vi "Part B.vi"() -> ()   [LabVIEW 2020]
uses:
  <vilib>/MakerHub/LINX/Public/Peripherals/Analog/Analog Read 1 Chan.vi
  <vilib>/MakerHub/LINX/Public/Peripherals/Digital/Digital Write N Chans.vi
  <vilib>/MakerHub/LINX/Public/Peripherals/Analog/Analog Read N Chans.vi
  <vilib>/MakerHub/LINX/Private/Local IO/LinxDigitalWrite.vi
  <vilib>/MakerHub/LINX/Public/Utilities/Check Channel.vi
  <vilib>/MakerHub/LINX/Private/Local IO/LinxAnalogRead.vi
  <vilib>/MakerHub/LINX/Public/Utilities/Open Serial.vi
  <vilib>/MakerHub/LINX/Private/Utilties/Generate Error.vi
  <vilib>/MakerHub/LINX/LMH-LINX.lvlib
panel:
  in  "?":bool
  out "Temp (C)":dbl(slide) scale=13.0..39.0
  out "Resistance of\nThermistor":dbl
  out "Voltage":dbl
  in  "Analog Channel":u8
  in  "Serial Port":refnum<visa-resource-name>="N/A"
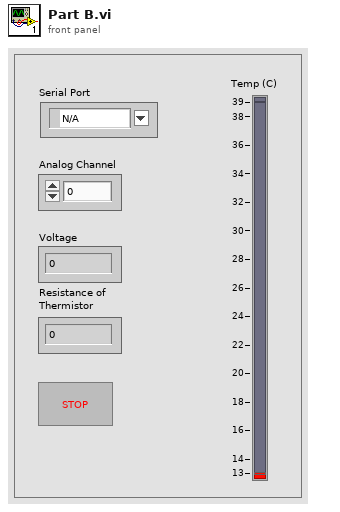
[diagram p1: front panel]
types:
  T1 = typedef "LMH-LINX.lvlib/LINX Ref.ctl" = cluster{"IO":T2, "Interface":T3, "LINX Device Config":T4}
  T2 = typedef "LMH-LINX.lvlib/Platform.ctl" = enum16{"Remote", "Local"}
  T3 = typedef "LMH-LINX.lvlib/Interface.ctl" = enum16{"Serial", "TCP"}
  T4 = typedef "LMH-LINX.lvlib/Device.lvlib/LINX Device Config.ctl" = cluster{"Interface":T3, "COM Port":refnum<visa-resource-name>, "TCP Configuration":T5, "Device Family":u8, "Device ID":u8, "Device Name":string, "TCP Ref":refnum<k5>, "Channels":T6}
  T5 = typedef "LMH-LINX.lvlib/Device.lvlib/TCP Config.ctl" = cluster{"IP Address":string, "Port":u16}
  T6 = typedef "LMH-LINX.lvlib/Channels.ctl" = cluster{"DI":u8[], "DO":u8[], "AI":u8[], "AO":u8[], "PWM":u8[], "QE":u8[], "UART":u8[], "I2C 2":u8[], "SPI":u8[], "CAN":u8[], "Servo":u8[], "AI Ref (V)":dbl, "AI Resolution (Bits)":u8, "AO Ref (V)":dbl, "AO Resolution (Bits)":u8}
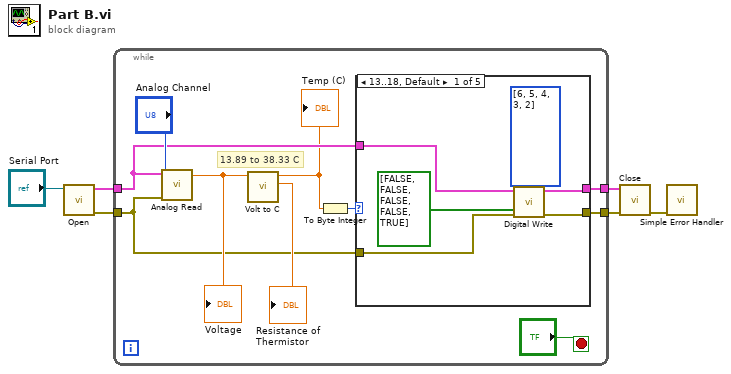
[diagram p0: block diagram]
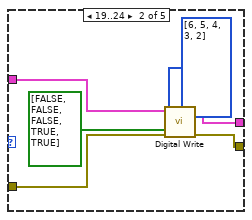
[diagram p2: hidden frame]
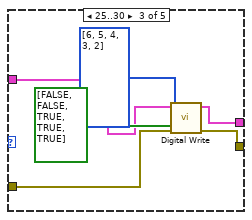
[diagram p3: hidden frame]
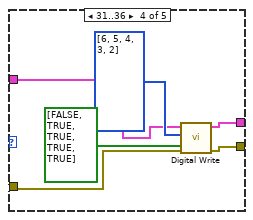
[diagram p4: hidden frame]
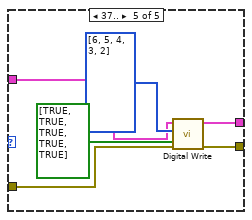
[diagram p5: hidden frame]
diagram:
  n1 = call-poly <vilib>:"Open.vi"("Serial Port"="Serial Port") -> ("Error Out"=w4:errorcluster, "LINX Resource"=w5:T1)  [unwired: 8 in, 1 out]
  n2 = while {
    tunnel: w5 -> [w12]
    tunnel: [w9] -> w2
    tunnel: w4 -> [w11]
    tunnel: [w8] -> w1
    stop <- "?" stop-if-true
    # "13.89 to 38.33 C"
    n3 = call-poly <vilib>:"Analog Read.vi"("Error In"=w11, "Analog Channel"="Analog Channel", "LINX Resource"=w12) -> ("Voltage"=w15:dbl)  [unwired: 5 in, 3 out]
    "Voltage" <- w15
    n4 = call "Volt to C.vi"("Voltage"=w15) -> ("R (ohm)"=→"Resistance of\nThermistor":dbl, "interpolation value"=w10:dbl)  [unwired: 9 in]
    "Temp (C)" <- w10
    n5 = To Byte Integer(number=w10) -> (8bit integer=w13:i8)
    n6 = case shown="13..18, Default" w13 {
      tunnel: [w21 w28 w33 w39 w45] -> w9
      tunnel: [w20 w27 w32 w38 w44] -> w8
      tunnel: w12 -> [w18 w24 w30 w36 w42]
      tunnel: w11 -> [w17 w23 w29 w35 w41]
      frame 13..18, Default {
        n7 = call-poly <vilib>:"Digital Write.vi"("Error In"=w17, "Values"=bool[] [FALSE, FALSE, FALSE, FALSE, TRUE], "DO Channels"=u8[] [6, 5, 4, 3, 2], "LINX Resource"=w18) -> ("Error Out"=w20:errorcluster, "LINX Resource"=w21:T1)  [unwired: 6 in]
      }
      frame 19..24 {
        n8 = call-poly <vilib>:"Digital Write.vi"("Error In"=w23, "Values"=bool[] [FALSE, FALSE, FALSE, TRUE, TRUE], "DO Channels"=u8[] [6, 5, 4, 3, 2], "LINX Resource"=w24) -> ("Error Out"=w27:errorcluster, "LINX Resource"=w28:T1)  [unwired: 6 in]
      }
      frame 25..30 {
        n9 = call-poly <vilib>:"Digital Write.vi"("Error In"=w29, "Values"=bool[] [FALSE, FALSE, TRUE, TRUE, TRUE], "DO Channels"=u8[] [6, 5, 4, 3, 2], "LINX Resource"=w30) -> ("Error Out"=w32:errorcluster, "LINX Resource"=w33:T1)  [unwired: 6 in]
      }
      frame 31..36 {
        n10 = call-poly <vilib>:"Digital Write.vi"("Error In"=w35, "Values"=bool[] [FALSE, TRUE, TRUE, TRUE, TRUE], "DO Channels"=u8[] [6, 5, 4, 3, 2], "LINX Resource"=w36) -> ("Error Out"=w38:errorcluster, "LINX Resource"=w39:T1)  [unwired: 6 in]
      }
      frame 37.. {
        n11 = call-poly <vilib>:"Digital Write.vi"("Error In"=w41, "Values"=bool[] [TRUE, TRUE, TRUE, TRUE, TRUE], "DO Channels"=u8[] [6, 5, 4, 3, 2], "LINX Resource"=w42) -> ("Error Out"=w44:errorcluster, "LINX Resource"=w45:T1)  [unwired: 6 in]
      }
    }
  }
  n12 = call <vilib>:"Close.vi"("Error In"=w1, "LINX Resource"=w2) -> ("Error Out"=w3:errorcluster)  [unwired: 9 in]
  n13 = call <vilib>:"Simple Error Handler.vi"("error in (no error)"=w3) -> ()  [unwired: 4 in, 5 out]
